vi "字符串链接数据库.vi"(8 "error in (no error)":errorcluster caption="错误输入（无错误）") -> (0 "error out":errorcluster caption="错误输出", 3 "连接字符串":string)   [LabVIEW 2013]
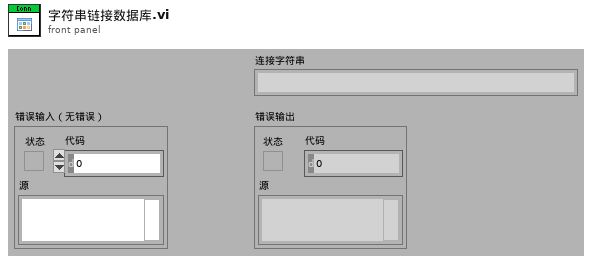
[diagram p1: front panel]
types:
  T1 = enum32{"invalid app kind", "Development System", "Run Time System", "Student Edition", "Embedded LabVIEW", "Evaluation", "Custom"}
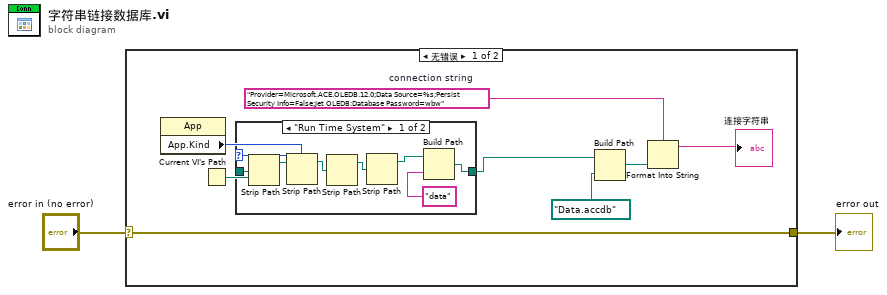
[diagram p0: block diagram]
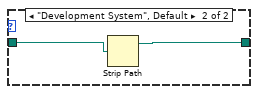
[diagram p2: hidden frame]
diagram:
  n1 = case shown="无错误" "error in (no error)" {
    selector: "error in (no error)" -> [w7 w20]
    tunnel: [w7 w20] -> w1
    frame No Error {
      w10 = "Provider=Microsoft.ACE.OLEDB.12.0;Data Source=%s;Persist Security Info=False;Jet OLEDB:Database Password=wbw"  # connection string
      n2 = property class="App"() -> ("App.Kind"=w5:T1)  [unwired: 2 in, 2 out]
      n3 = Current VI's Path() -> (path=w6:path)
      n4 = case shown="\"Run Time System\"" w5 {
        tunnel: w6 -> [w17 w19]
        tunnel: [w15 w18] -> w4
        frame "Run Time System" {
          n5 = Strip Path(path=w17) -> (stripped path=w14:path)  [unwired: 1 out]
          n6 = Strip Path(path=w14) -> (stripped path=w13:path)  [unwired: 1 out]
          n7 = Strip Path(path=w13) -> (stripped path=w12:path)  [unwired: 1 out]
          n8 = Strip Path(path=w12) -> (stripped path=w11:path)  [unwired: 1 out]
          n9 = Build Path(base path=w11, name or relative path="data" ("名称或相对路径")) -> (appended path=w15:path)
        }
        frame "Development System", Default {
          n10 = Strip Path(path=w19) -> (stripped path=w18:path)  [unwired: 1 out]
        }
      }
      n11 = Build Path(base path=w4, name or relative path=path "Data.accdb" ("名称或相对路径")) -> (appended path=w9:path)
      n12 = Format Into String(format string=w10, w9) -> (resulting string=→"连接字符串":string)  [unwired: 2 in, 1 out]
    }
    frame Error {
    }
  }
  "error out" <- w1
